vi "获取一个图像区域的信息.vi"(10 "Img in":T1, 11 "Results (端子弹片)":string[][](array[string])) -> (0 "区域标准差":dbl[](array[numeric]), 1 "区域亮度平均值":dbl[](array[numeric]), 2 "矩形框":dbl[][](array[numeric]), 3 "所有信息":dbl[][](array[numeric]))   [LabVIEW 2014]
uses:
  <vilib>/vision/Image Controls.llb/IMAQ Image.ctl
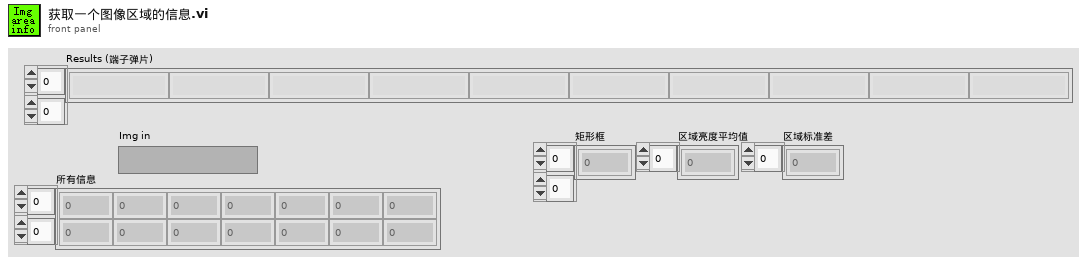
[diagram p1: front panel]
types:
  T1 = typedef "IMAQ Image.ctl" = refnum<image>
  T2 = cluster{"[0]":dbl, "[1]":dbl, "[2]":dbl, "[3]":dbl}
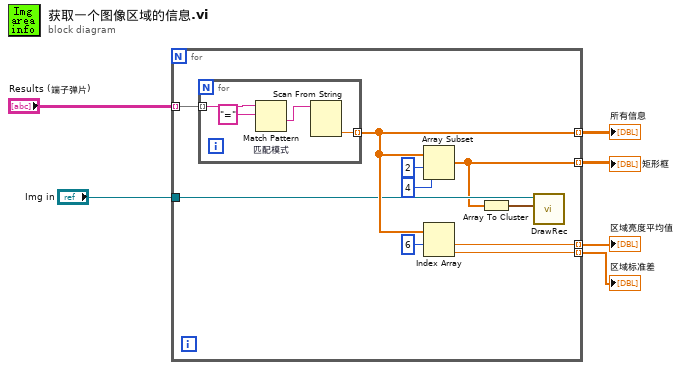
[diagram p0: block diagram]
diagram:
  n1 = for {
    tunnel: "Results (端子弹片)" -> [w16] mode=indexing
    tunnel: [w13] -> w6 mode=indexing
    tunnel: [w7] -> w4 mode=indexing
    tunnel: [w12] -> w3 mode=indexing
    tunnel: [w10] -> w2 mode=indexing
    tunnel: "Img in" -> [w8]
    n2 = for {
      tunnel: w16 -> [w19] mode=indexing
      tunnel: [w17] -> w13 mode=indexing
      n3 = Match Pattern "匹配模式"(string=w19, regular expression="=" ("搜索字符串")) -> (after substring=w18:string)  [unwired: 1 in, 3 out]
      n4 = Scan From String(input string=w18) -> (output 1=w17:dbl)  [unwired: 4 in, 3 out]
    }
    n5 = Array Subset(array=w13, index=2 ("索引"), length=4 ("长度")) -> (w7:dbl[])
    n6 = Index Array(array=w13, index #1=6 ("索引")) -> (element #1=w12:dbl, element #2=w10:dbl)  [unwired: 1 in]
    n7 = Array To Cluster(array=w7) -> (cluster=w9:T2)
    n8 = call "DrawRec.vi"("Rectangle"=w9, "Image"=w8) -> ()  [unwired: 9 in, 1 out]
  }
  "所有信息" <- w6
  "矩形框" <- w4
  "区域亮度平均值" <- w3
  "区域标准差" <- w2
